vi "Wait to use camera - SubVI.vi"(1 "error in":errorcluster) -> (0 "error out":errorcluster)   [LabVIEW 2014]
uses:
  camera globals - SubVI.vi
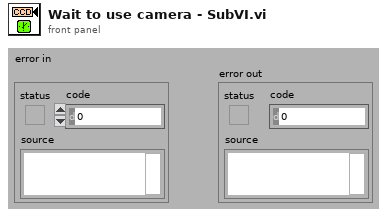
[diagram p1: front panel]
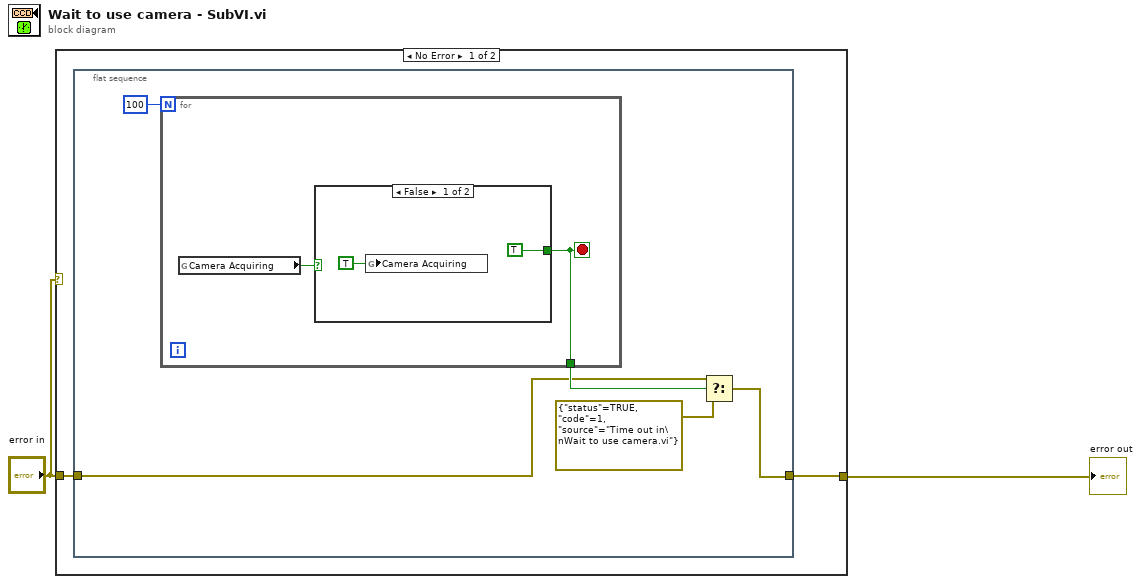
[diagram p0: block diagram]
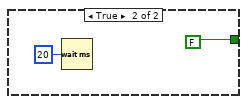
[diagram p2: hidden frame]
diagram:
  n1 = case shown="No Error" "error in" {
    tunnel: [w4 w16] -> w2
    tunnel: "error in" -> [w3 w16]
    frame No Error {
      n2 = flat-sequence {
        tunnel: w3 -> [w6]
        tunnel: [w8] -> w4
        frame #0 {
          n3 = for {
            N: 100 ("Numeric") -> [_]
            tunnel: [w10] -> w7
            stop <- w10 stop-if-true
            n4 = global read "camera globals - SubVI.vi" "Camera Acquiring"() -> (w11:bool)
            n5 = case shown="False" w11 {
              tunnel: [TRUE FALSE] -> w10
              frame False {
                n6 = global write "camera globals - SubVI.vi" "Camera Acquiring"(TRUE ("Camera Acquiring")) -> ()
              }
              frame True {
                n7 = Wait (ms)(milliseconds to wait=u32 20) -> ()  [unwired: 1 out]
              }
            }
          }
          n8 = Select(t=w6, s=w7, f=errorcluster {"status"=TRUE, "code"=1, "source"="Time out in\nWait to use camera.vi"}) -> (s? t:f=w8:errorcluster)
        }
      }
    }
    frame Error {
    }
  }
  "error out" <- w2
